vi "Run Framework.vi"(5 "components directory":path, 7 "framework options":T14={"FIFO Options"={"Infinite Timeouts"=FALSE}, "Thread Options"={"Show FP On Call"=TRUE, "Close FP After Call"=TRUE, "Allow Debugging"=TRUE, "Restart On Error"=FALSE}, "Plugin Options"={"Default Components"=TRUE}, "Performance Options"={"Measure Period"=TRUE, "Measure Rx/Tx Duration"=TRUE}}, 8 "error in (no error)":errorcluster, 9 "thread settings":cluster{"Processor":i32, "Priority":i32}={"Processor"=-2, "Priority"=100}, 10 "framework configuration":T2, 11 "user interface pointers (null)":T1) -> (0 "error out":errorcluster)   [LabVIEW 2017]
uses:
  Classes/Framework/Framework Options.ctl
  Typedefs/DSF FIFO Options.ctl
  Classes/Thread/Thread Options.ctl
  Typedefs/DSF Plugin Options.ctl
  Typedefs/DSF Performance Options.ctl
  Typedefs/DSF Engine Framework Configuration.ctl
  Typedefs/DSF Engine Plugin Configuration.ctl
  Typedefs/DSF Timing Info.ctl
  Typedefs/DSF Engine Plugin Thread Configuration.ctl
  Typedefs/DSF Settings Info.ctl
  Typedefs/DSF Engine Transfer Group Configuration.ctl
  Typedefs/DSF Direction.ctl
  Typedefs/DSF Engine Transfer Configuration.ctl
  Typedefs/DSF Byte Order.ctl
  Typedefs/DSF Engine Channel Configuration.ctl
  Typedefs/DSF Data Type.ctl
  Typedefs/DSF Timeout Behavior.ctl
  Typedefs/DSF UI Pointers.ctl
  <vilib>/NI/Memory Manager/Classes/Pointer/Pointer.lvclass
  <vilib>/NI/Memory Manager/Classes/Pointer/Pointer.lvclass/Pointer.ctl
  <vilib>/Platform/TimedLoop/XDataNode/timing_clust.ctl
  <vilib>/Platform/TimedLoop/XDataNode/nitl_modes.ctl
  <vilib>/Platform/TimedLoop/XDataNode/wakeup.ctl
  <vilib>/NI/Memory Manager/Classes/Pointer/Write U32.vi
  <vilib>/NI/Memory Manager/Classes/Pointer/Read U32.vi
  <vilib>/NI/Memory Manager/Classes/Pointer/Read I32.vi
  <vilib>/NI/Memory Manager/Classes/Pointer/Read Bool.vi
  <vilib>/NI/Memory Manager/Classes/Pointer/Write Bool.vi
  <vilib>/NI/Memory Manager/Classes/Pointer/Write I32.vi
  <vilib>/NI/Memory Manager/Classes/Pointer/Set Address.vi
  <vilib>/NI/Memory Manager/Classes/Pointer/Set Size.vi
  <vilib>/NI/Memory Manager/Classes/Pointer/Set Internal.vi
  <vilib>/NI/Memory Manager/Classes/Pointer/Check Null Pointer.vi
  <vilib>/NI/Memory Manager/Classes/Pointer/Clear (No Check).vi
  <vilib>/NI/Memory Manager/Classes/Pointer/Check Length.vi
  <vilib>/NI/Memory Manager/Classes/Pointer/Write (No Check).vi
  <vilib>/NI/Memory Manager/Classes/Pointer/Write (No Check) U32.vi
  <vilib>/NI/Memory Manager/Classes/Pointer/Check Move.vi
  <vilib>/NI/Memory Manager/Classes/Pointer/Read (No Check).vi
  <vilib>/NI/Memory Manager/Classes/Pointer/Read (No Check) U32.vi
  <vilib>/NI/Memory Manager/Classes/Pointer/Read (No Check) I32.vi
  <vilib>/NI/Memory Manager/Classes/Pointer/Read (No Check) Bool.vi
  <vilib>/NI/Memory Manager/Classes/Pointer/Write (No Check) Bool.vi
  <vilib>/NI/Memory Manager/Classes/Pointer/Write (No Check) I32.vi
  <vilib>/NI/Memory Manager/Classes/Pointer/Get Internal.vi
  <vilib>/NI/Memory Manager/Classes/Pointer/Errors.vi
  <vilib>/NI/Memory Manager/Classes/Pointer/Zone.vi
  <vilib>/NI/Memory Manager/Classes/Pointer/Null Pointer.vi
  <vilib>/NI/Memory Manager/Classes/Pointer/Check Bounds (Pointer).vi
  <vilib>/NI/Memory Manager/Classes/Pointer/Check Count.vi
  <vilib>/NI/Memory Manager/Classes/Pointer/Check Bounds (Power of 2).vi
  <vilib>/NI/Memory Manager/Classes/Pointer/Create Error.vi
  <vilib>/NI/Memory Manager/Classes/Pointer/Out of Bounds.vi
  <vilib>/NI/Memory Manager/Classes/Pointer/Check Bounds.vi
  <vilib>/NI/Memory Manager/Constants/Constants.vi
  <vilib>/NI/Memory Manager/Constants/Library Name.vi
  <vilib>/NI/Memory Manager/Classes/Pointer/Pointer Error Info.vi
  <vilib>/NI/Memory Manager/Constants/Pointer Class Name.vi
  <vilib>/NI/Memory Manager/Classes/Pointer/Write Pointer Size to Error.vi
  <vilib>/NI/Memory Manager/Classes/Pointer/Check Bounds (Buffer).vi
  <vilib>/NI/Memory Manager/Classes/Pointer/Buffer Underflow.vi
  <vilib>/NI/Memory Manager/VIs/New Error Cluster.vi
  <vilib>/NI/Memory Manager/VIs/New Error Cluster (512B).vi
  <vilib>/NI/Memory Manager/VIs/Set Error Status.vi
  <vilib>/NI/Memory Manager/VIs/Set Error Code.vi
  <vilib>/NI/Memory Manager/VIs/Set Error Source.vi
  <vilib>/NI/Memory Manager/VIs/Write String to Source.vi
  <vilib>/NI/Memory Manager/VIs/Write Numeric to Source.vi
  <vilib>/NI/Memory Manager/VIs/Write Numeric Scalar to Source (Base10 U64).vi
  Classes/Framework/Framework.lvclass
  <vilib>/platform/TimedLoop/XDataNode/XDataNode.xnode
  <vilib>/Platform/TimedLoop/XDataNode/XDNodeRunTimeDep.lvlib
  DSF Core.lvlib
  Classes/Thread/Thread.lvclass
panel:
  out "actual frequency":u32 format="%.0pHz"
  in  "target frequency":u32=100 format="%.0pHz"
  out "iteration":i32
  in  "stop":bool
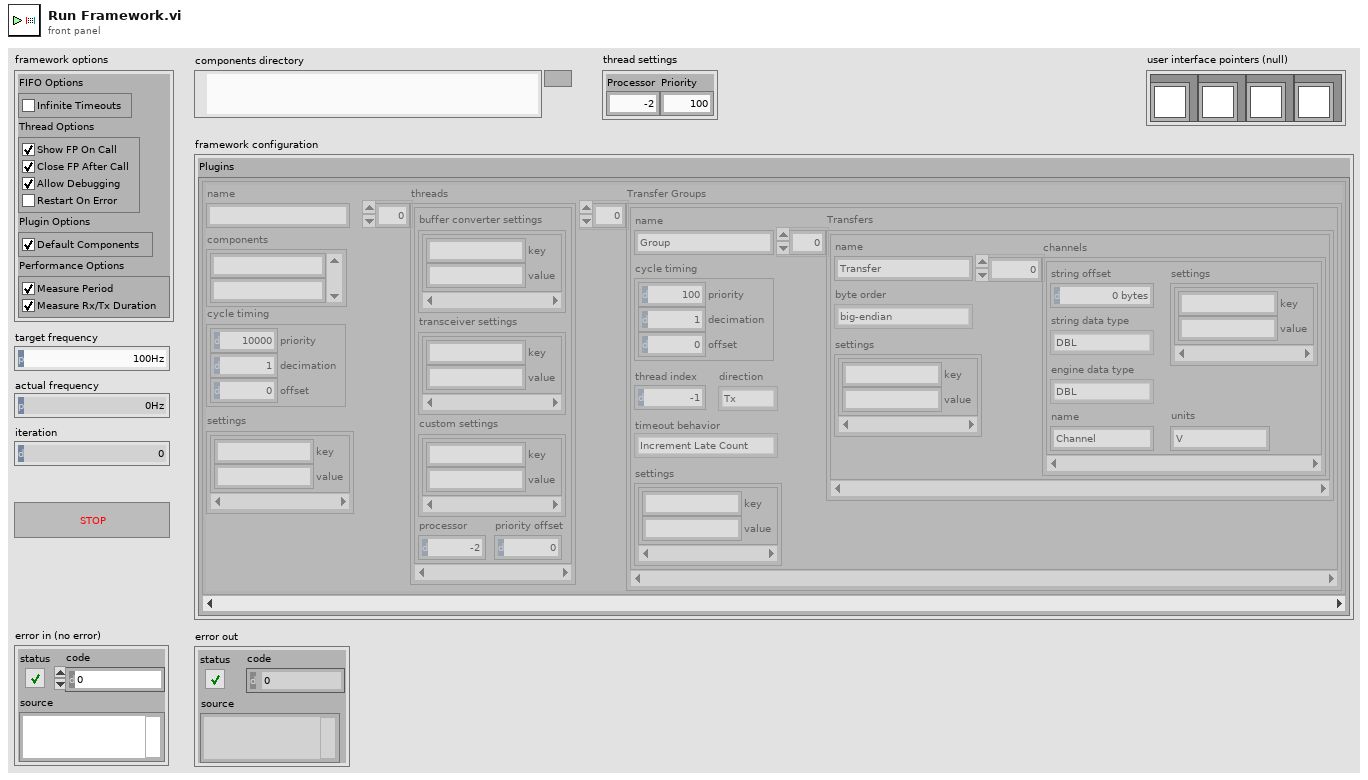
[diagram p1: front panel]
types:
  T1 = typedef "DSF Core.lvlib/DSF UI Pointers.ctl" = cluster{"Stop":refnum<class "Pointer.lvclass">, "Target Period":refnum<class "Pointer.lvclass">, "Actual Period":refnum<class "Pointer.lvclass">, "Iteration":refnum<class "Pointer.lvclass">}
  T2 = typedef "DSF Core.lvlib/DSF Engine Framework Configuration.ctl" = cluster{"Plugins":T3[]}
  T3 = typedef "DSF Core.lvlib/DSF Engine Plugin Configuration.ctl" = cluster{"name":string, "components":string[], "cycle timing":T4, "threads":T5[], "Transfer Groups":T7[], "settings":T6}
  T4 = typedef "DSF Core.lvlib/DSF Timing Info.ctl" = cluster{"priority":u64, "decimation":u64, "offset":u64}
  T5 = typedef "DSF Core.lvlib/DSF Engine Plugin Thread Configuration.ctl" = cluster{"buffer converter settings":T6, "transceiver settings":T6, "custom settings":T6, "processor":i32, "priority offset":i16}
  T6 = typedef "DSF Core.lvlib/DSF Settings Info.ctl" = cluster{"key":string, "value":string}[]
  T7 = typedef "DSF Core.lvlib/DSF Engine Transfer Group Configuration.ctl" = cluster{"name":string, "direction":T8, "cycle timing":T4, "thread index":i32, "settings":T6, "Transfers":T9[], "timeout behavior":T13}
  T8 = typedef "DSF Core.lvlib/DSF Direction.ctl" = enum8{"Tx", "Rx"}
  T9 = typedef "DSF Core.lvlib/DSF Engine Transfer Configuration.ctl" = cluster{"name":string, "byte order":T10, "settings":T6, "channels":T11[]}
  T10 = typedef "DSF Core.lvlib/DSF Byte Order.ctl" = enum8{"big-endian", "little-endian"}
  T11 = typedef "DSF Core.lvlib/DSF Engine Channel Configuration.ctl" = cluster{"string offset":u64, "string data type":T12, "engine data type":T12, "name":string, "settings":T6, "units":string}
  T12 = typedef "DSF Core.lvlib/DSF Data Type.ctl" = enum8{"Bool", "SGL", "DBL", "I8", "I16", "I32", "I64", "U8", "U16", "U32", "U64"}
  T13 = typedef "DSF Core.lvlib/DSF Timeout Behavior.ctl" = enum8{"Increment Late Count", "Throw Error"}
  T14 = typedef "DSF Core.lvlib/Framework.lvclass/Framework Options.ctl" = cluster{"FIFO Options":T15, "Thread Options":T16, "Plugin Options":T17, "Performance Options":T18}
  T15 = typedef "DSF Core.lvlib/Framework.lvclass/DSF FIFO Options.ctl" = cluster{"Infinite Timeouts":bool}
  T16 = typedef "DSF Core.lvlib/Thread.lvclass/Thread Options.ctl" = cluster{"Show FP On Call":bool, "Close FP After Call":bool, "Allow Debugging":bool, "Restart On Error":bool}
  T17 = typedef "DSF Core.lvlib/Framework.lvclass/DSF Plugin Options.ctl" = cluster{"Default Components":bool}
  T18 = typedef "DSF Core.lvlib/DSF Performance Options.ctl" = cluster{"Measure Period":bool, "Measure Rx/Tx Duration":bool}
  T19 = typedef "XDNodeRunTimeDep.lvlib/timing_clust.ctl" = cluster{"Expected End [f-1]":u64, "Actual End [f-1]":u64, "Finished Late? [f-1]":bool, "Expected End [i-1]":u64, "Actual End [i-1]":u64, "Finished Late? [i-1]":bool, "Expected Start [i]":u64, "Actual Start [i]":u64, "Expected Start [f]":u64, "Actual Start [f]":u64, "Source Name":string, "Structure Name":string, "Period":i64, "Deadline":i64, "Offset":i64, "Start":i64, "Priority":i32, "Timeout":i32, "Mode":T20, "Wakeup Reason":T21, "Error":errorcluster, "Source Type":string, "Secondary Source Type":string, "Global End Time":u64, "Global Start Time":u64, "Frame Duration":u64, "Iteration Duration":u64, "Assigned CPU":i32, "I/O Scan Engine Mode":u32}
  T20 = typedef "XDNodeRunTimeDep.lvlib/nitl_modes.ctl" = enum32{"No Change", "Process missed periods, maintain original phase", "Discard missed periods, maintain original phase", "Process missed periods, ignore original phase", "Discard missed periods, ignore original phase"}
  T21 = typedef "XDNodeRunTimeDep.lvlib/wakeup.ctl" = enum32{"Normal", "Aborted", "Asynchronous wakeup", "Timing source error", "Timed loop error", "Timeout"}
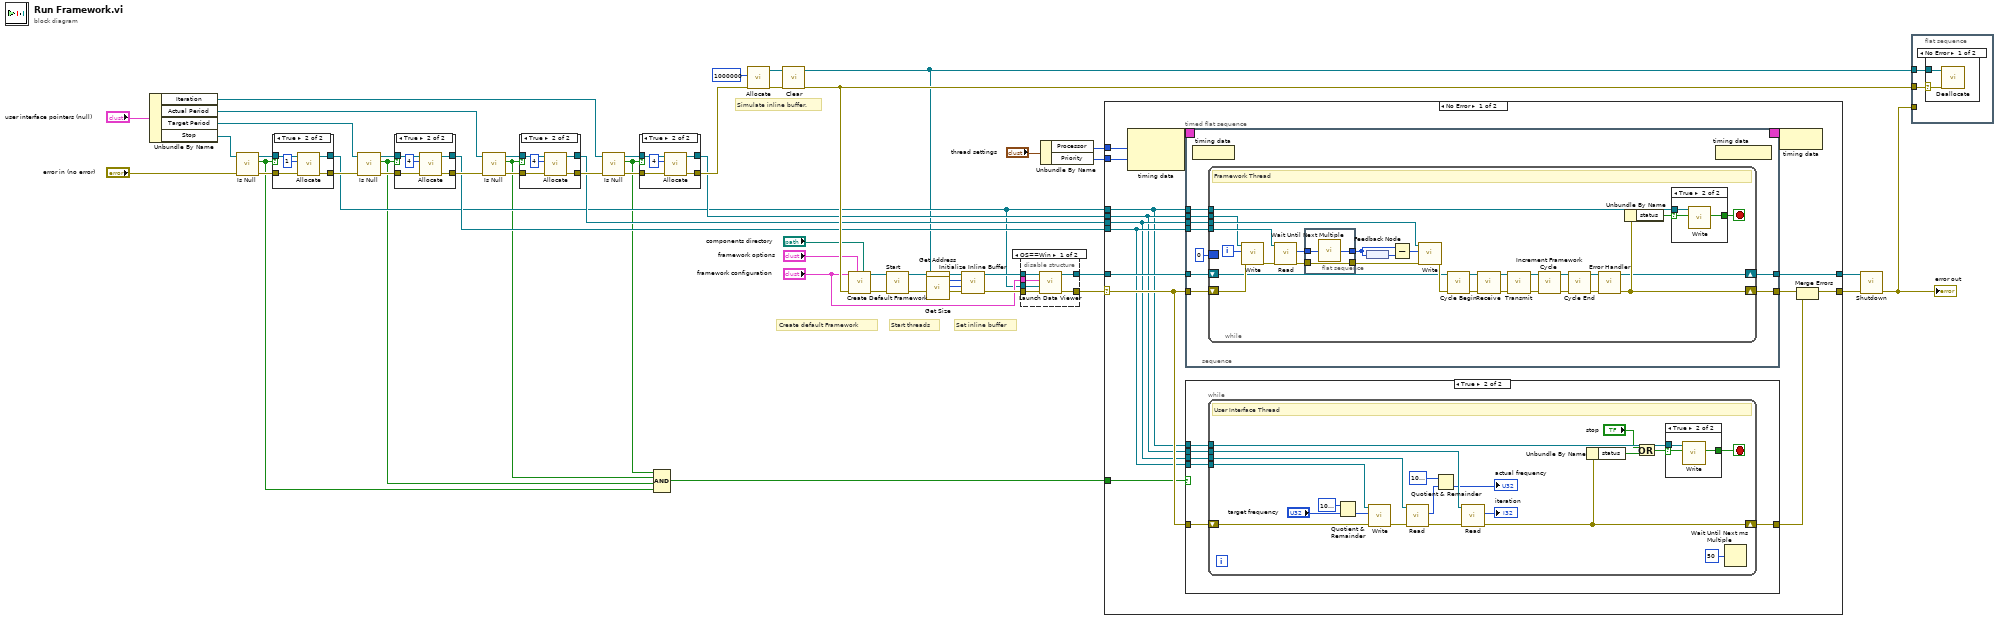
[diagram p0: block diagram]
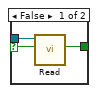
[diagram p5: hidden frame]
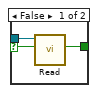
[diagram p6: hidden frame]
diagram:
  # "Set inline buffer"
  # "Start threads"
  # "Create default Framework"
  # "Simulate inline buffer."
  n1 = Unbundle By Name("user interface pointers (null)") -> ("Iteration"=w18:refnum<class "Pointer.lvclass">, "Actual Period"=w22:refnum<class "Pointer.lvclass">, "Target Period"=w26:refnum<class "Pointer.lvclass">, "Stop"=w32:refnum<class "Pointer.lvclass">)
  n2 = call <vilib>:"Is Null.vi"("error in (no error)"="error in (no error)", "Pointer in"=w32) -> ("error out"=w30:errorcluster, "null?"=w5:bool, "Pointer out"=w31:refnum<class "Pointer.lvclass">)  [unwired: 7 in]
  n3 = case shown="True" w5 {
    tunnel: w31 -> [w53 w57]
    tunnel: w30 -> [w52 w56]
    tunnel: [w53 w55] -> w11
    tunnel: [w52 w54] -> w27
    frame False {
    }
    frame True {
      n4 = call <vilib>:"Allocate.vi"("error in (no error)"=w56, "size"=u64 1, "Pointer type"=w57) -> ("error out"=w54:errorcluster, "Pointer out"=w55:refnum<class "Pointer.lvclass">)  [unwired: 7 in]
    }
  }
  n5 = call <vilib>:"Is Null.vi"("error in (no error)"=w27, "Pointer in"=w26) -> ("error out"=w28:errorcluster, "null?"=w4:bool, "Pointer out"=w29:refnum<class "Pointer.lvclass">)  [unwired: 7 in]
  n6 = case shown="True" w4 {
    tunnel: w29 -> [w60 w64]
    tunnel: w28 -> [w59 w63]
    tunnel: [w60 w62] -> w16
    tunnel: [w59 w61] -> w23
    frame False {
    }
    frame True {
      n7 = call <vilib>:"Allocate.vi"("error in (no error)"=w63, "size"=u64 4, "Pointer type"=w64) -> ("error out"=w61:errorcluster, "Pointer out"=w62:refnum<class "Pointer.lvclass">)  [unwired: 7 in]
    }
  }
  n8 = call <vilib>:"Is Null.vi"("error in (no error)"=w23, "Pointer in"=w22) -> ("error out"=w24:errorcluster, "null?"=w3:bool, "Pointer out"=w25:refnum<class "Pointer.lvclass">)  [unwired: 7 in]
  n9 = case shown="True" w3 {
    tunnel: w25 -> [w67 w71]
    tunnel: w24 -> [w66 w70]
    tunnel: [w67 w69] -> w13
    tunnel: [w66 w68] -> w19
    frame False {
    }
    frame True {
      n10 = call <vilib>:"Allocate.vi"("error in (no error)"=w70, "size"=u64 4, "Pointer type"=w71) -> ("error out"=w68:errorcluster, "Pointer out"=w69:refnum<class "Pointer.lvclass">)  [unwired: 7 in]
    }
  }
  n11 = call <vilib>:"Is Null.vi"("error in (no error)"=w19, "Pointer in"=w18) -> ("error out"=w20:errorcluster, "null?"=w2:bool, "Pointer out"=w21:refnum<class "Pointer.lvclass">)  [unwired: 7 in]
  n12 = case shown="True" w2 {
    tunnel: w21 -> [w74 w78]
    tunnel: w20 -> [w73 w77]
    tunnel: [w74 w76] -> w14
    tunnel: [w73 w75] -> w17
    frame False {
    }
    frame True {
      n13 = call <vilib>:"Allocate.vi"("error in (no error)"=w77, "size"=u64 4, "Pointer type"=w78) -> ("error out"=w75:errorcluster, "Pointer out"=w76:refnum<class "Pointer.lvclass">)  [unwired: 7 in]
    }
  }
  n14 = Compound Arithmetic op=AND(w2, w3, w4, w5) -> (w1:bool)
  n15 = call <vilib>:"Allocate.vi"("error in (no error)"=w17, "size"=u64 1000000) -> ("error out"=w46:errorcluster, "Pointer out"=w43:refnum<class "Pointer.lvclass">)  [unwired: 8 in]
  n16 = call <vilib>:"Clear.vi"("error in (no error)"=w46, "Pointer in"=w43) -> ("error out"=w51:errorcluster, "Pointer out"=w10:refnum<class "Pointer.lvclass">)  [unwired: 8 in]
  n17 = call "Create Default Framework.vi"("components directory (default)"="components directory", "framework options"="framework options", "error in (no error)"=w51, "framework configuration"="framework configuration") -> ("error out"=w38:errorcluster, "Framework"=w42:refnum<class "Framework.lvclass">)  [unwired: 6 in]
  n18 = call-dynamic "Start.vi"("error in (no error)"=w38, "Framework in"=w42) -> ("error out"=w41:errorcluster, "Framework out"=w50:refnum<class "Framework.lvclass">)  [unwired: 8 in]
  n19 = call <vilib>:"Get Address.vi"("Pointer in"=w10) -> ("address"=w44:u64)  [unwired: 9 in, 1 out]
  n20 = call <vilib>:"Get Size.vi"("Pointer in"=w10) -> ("size"=w45:u64)  [unwired: 9 in, 1 out]
  n21 = call "Initialize Inline Buffer.vi"("error in (no error)"=w41, "size"=w45, "address"=w44, "Framework in"=w50) -> ("error out"=w39:errorcluster, "Framework out"=w40:refnum<class "Framework.lvclass">)  [unwired: 6 in]
  n22 = disable-structure shown="OS==Win" {
    disable-tunnel: [w85 w87] -> w36
    disable-tunnel: [w84 w86] -> w15
    disable-tunnel: w40 -> [w83 w87]
    disable-tunnel: w39 -> [w82 w86]
    disable-tunnel: "framework configuration" -> [w81 _]
    disable-tunnel: w11 -> [w80 _]
    frame condition #0 (active) {
      n23 = call "Launch Data Viewer.vi"("error in (no error)"=w82, "Stop Pointer"=w80, "Framework Configuration"=w81, "Framework in"=w83) -> ("error out"=w84:errorcluster, "Framework out"=w85:refnum<class "Framework.lvclass">)  [unwired: 6 in]
    }
    frame condition #1 {
    }
  }
  n24 = Unbundle By Name("thread settings") -> ("Processor"=w7:i32, "Priority"=w8:i32)
  n25 = case shown="No Error" w15 {
    selector: w15 -> [w102 w198]
    tunnel: [w95 w198] -> w49
    tunnel: w36 -> [w101 w199]
    tunnel: [w99 w199] -> w48
    tunnel: w11 -> [w92 _]
    tunnel: w16 -> [w100 _]
    tunnel: w13 -> [w94 _]
    tunnel: w14 -> [w93 _]
    tunnel: w7 -> [w91 _]
    tunnel: w8 -> [w90 _]
    tunnel: w1 -> [w89 _]
    frame No Error {
      n26 = node-c288(w91, w90) -> (w98:T19)
      n27 = timed-sequence {
        timing: w98 -> [_]
        timing-out: [_] -> w97
        tunnel: w101 -> [w143]
        tunnel: w102 -> [w142]
        tunnel: [w141] -> w99
        tunnel: [w140] -> w96
        tunnel: w92 -> [w139]
        tunnel: w100 -> [w138]
        tunnel: w94 -> [w137]
        tunnel: w93 -> [w136]
        n28 = timed-flat-sequence {
          tunnel: w143 -> [w152]
          tunnel: w142 -> [w151]
          tunnel: [w150] -> w141
          tunnel: [w149] -> w140
          tunnel: w139 -> [w148]
          tunnel: w138 -> [w147]
          tunnel: w137 -> [w146]
          tunnel: w136 -> [w145]
          n29 = node-c288() -> ()  [unwired: 1 in]
          n30 = while {
            shift-right: [w171] -> w150
            shift-left: w152 -> [w156]
            tunnel: w148 -> [w179]
            shift-right: [w174] -> w149
            shift-left: w151 -> [w160]
            tunnel: w147 -> [w172]
            tunnel: w146 -> [w162]
            tunnel: w145 -> [w159]
            border: u32 0 ("Tick Count(uSec)") -> [_]
            i -> [w164]
            stop <- w178 stop-if-true
            # "Framework Thread"
            n31 = call-poly <vilib>:"Write.vi"("error in (no error)"=w160, "value"=w164, "Pointer in"=w159) -> ("error out"=w161:errorcluster)  [unwired: 5 in, 3 out]
            n32 = call-poly <vilib>:"Read.vi"("error in (no error)"=w161, "Pointer in"=w172) -> ("error out"=w158:errorcluster, "value out"=w173:u32)  [unwired: 6 in, 2 out]
            n33 = flat-sequence {
              tunnel: w173 -> [w184]
              tunnel: [w183] -> w155
              tunnel: w158 -> [w182]
              tunnel: [w182] -> w157
              frame #0 {
                n34 = call "Wait Until Next Multiple"("Count(uSec)"=w184) -> ("Tick Count(uSec)"=w183:u32)
              }
            }
            n35 = feedback-in #1(w155) -> ()
            n36 = feedback #1() -> (w153:u32)
            n37 = Subtract(x=w155, y=w153) -> (x-y=w154:u32)
            n38 = call-poly <vilib>:"Write.vi"("error in (no error)"=w157, "value"=w154, "Pointer in"=w162) -> ("error out"=w163:errorcluster)  [unwired: 5 in, 3 out]
            n39 = call "Cycle Begin.vi"("error in (no error)"=w163, "Framework in"=w156) -> ("error out"=w176:errorcluster, "Framework out"=w177:refnum<class "Framework.lvclass">)  [unwired: 8 in]
            n40 = call "Receive.vi"("error in (no error)"=w176, "Framework in"=w177) -> ("error out"=w181:errorcluster, "Framework out"=w180:refnum<class "Framework.lvclass">)  [unwired: 8 in]
            n41 = call "Transmit.vi"("error in (no error)"=w181, "Framework in"=w180) -> ("error out"=w170:errorcluster, "Framework out"=w169:refnum<class "Framework.lvclass">)  [unwired: 8 in]
            n42 = call "Increment Framework Cycle.vi"("error in (no error)"=w170, "Framework in"=w169) -> ("error out"=w167:errorcluster, "Framework out"=w168:refnum<class "Framework.lvclass">)  [unwired: 8 in]
            n43 = call "Cycle End.vi"("error in (no error)"=w167, "Framework in"=w168) -> ("error out"=w166:errorcluster, "Framework out"=w165:refnum<class "Framework.lvclass">)  [unwired: 8 in]
            n44 = call "Error Handler.vi"("error in (no error)"=w166, "Framework in"=w165) -> ("error out"=w174:errorcluster, "Framework out"=w171:refnum<class "Framework.lvclass">)  [unwired: 8 in]
            n45 = Unbundle By Name(w174) -> ("status"=w175:bool)
            n46 = case shown="True" w175 {
              selector: w175 -> [w186 w189]
              tunnel: w179 -> [w187 w190]
              tunnel: [w185 w188] -> w178
              frame False {
                n47 = call-poly <vilib>:"Read.vi"("value in"=w186, "Pointer in"=w187) -> ("value out"=w185:bool)  [unwired: 6 in, 3 out]
              }
              frame True {
                n48 = call-poly <vilib>:"Write.vi"("value"=w189, "Pointer in"=w190) -> ("value"=w188:bool)  [unwired: 6 in, 3 out]
              }
            }
          }
          n49 = node-c288() -> ()  [unwired: 1 out]
        }
      }
      n50 = case shown="True" w89 {
        tunnel: w102 -> [w103 w109]
        tunnel: w100 -> [_ w108]
        tunnel: [w103 w107] -> w88
        tunnel: w94 -> [_ w106]
        tunnel: w93 -> [_ w105]
        tunnel: w92 -> [_ w104]
        frame False {
        }
        frame True {
          n51 = while {
            tunnel: w104 -> [w129]
            shift-right: [w116] -> w107
            shift-left: w109 -> [w124]
            tunnel: w108 -> [w120]
            tunnel: w106 -> [w118]
            tunnel: w105 -> [w114]
            stop <- w128 stop-if-true
            # "User Interface Thread"
            n52 = Quotient & Remainder(x=u32 1000000 ("y"), y="target frequency") -> (floor(x/y)=w119:u32)  [unwired: 1 out]
            n53 = call-poly <vilib>:"Write.vi"("error in (no error)"=w124, "value"=w119, "Pointer in"=w120) -> ("error out"=w121:errorcluster)  [unwired: 5 in, 3 out]
            n54 = call-poly <vilib>:"Read.vi"("error in (no error)"=w121, "Pointer in"=w118) -> ("error out"=w117:errorcluster, "value out"=w110:u32)  [unwired: 6 in, 2 out]
            n55 = Quotient & Remainder(x=u32 1000000 ("y"), y=w110) -> (floor(x/y)=→"actual frequency":u32)  [unwired: 1 out]
            n56 = call-poly <vilib>:"Read.vi"("error in (no error)"=w117, "Pointer in"=w114) -> ("error out"=w116:errorcluster, "value out"=→"iteration":i32)  [unwired: 6 in, 2 out]
            n57 = Unbundle By Name(w116) -> ("status"=w126:bool)
            n58 = Or(x="stop", y=w126) -> (x .or. y?=w127:bool)
            n59 = case shown="True" w127 {
              selector: w127 -> [w131 w134]
              tunnel: w129 -> [w132 w135]
              tunnel: [w130 w133] -> w128
              frame False {
                n60 = call-poly <vilib>:"Read.vi"("value in"=w131, "Pointer in"=w132) -> ("value out"=w130:bool)  [unwired: 6 in, 3 out]
              }
              frame True {
                n61 = call-poly <vilib>:"Write.vi"("value"=w134, "Pointer in"=w135) -> ("value"=w133:bool)  [unwired: 6 in, 3 out]
              }
            }
            n62 = Wait Until Next ms Multiple(millisecond multiple=u32 50) -> ()  [unwired: 1 out]
          }
        }
      }
      n63 = node-c288(w97) -> ()
      n64 = Merge Errors(w96, w88) -> (w95:errorcluster)
    }
    frame Error {
    }
  }
  n65 = call-dynamic "Shutdown.vi"("error in (no error)"=w49, "Framework in"=w48) -> ("error out"=w37:errorcluster)  [unwired: 8 in, 1 out]
  "error out" <- w37
  n66 = flat-sequence {
    tunnel: w10 -> [w201]
    tunnel: w37 -> [_]
    tunnel: w51 -> [w200]
    frame #0 {
      n67 = case shown="No Error" w200 {
        selector: w200 -> [w202 _]
        tunnel: w201 -> [w203 _]
        frame No Error {
          n68 = call <vilib>:"Deallocate.vi"("error in (no error)"=w202, "Pointer"=w203) -> ()  [unwired: 8 in, 2 out]
        }
        frame Error {
        }
      }
    }
  }
